vi "Frame.Export.vi"(8 "error in (no error)":errorcluster, 11 "Item Ref in":T1 format="%.0x") -> (0 "error out":errorcluster, 2 "Frame":T2 {"Signals"."Byte Order" items=["Little Endian", "Big Endian"]; "Signals"."Data Type" items=["Signed", "Unsigned", "IEEE Float"]}, 3 "Item Ref out":T1 format="%.0x")   [LabVIEW 2015, in "Diagnostics Addon System Explorer.lvlib"]
uses:
  Diagnostics Addon System Explorer.lvlib
  Types/Frame.Export.ctl
  Shared/Types/Signal.ctl
  <vilib>/NI Veristand/Custom Device API/Custom Device Item Ref.ctl
  Types/FG.Action.ctl
  Signal.FG.vi
  <vilib>/NI Veristand/Custom Device API/NI VeriStand - Get Custom Device Channel Data.vi
  <vilib>/NI Veristand/Custom Device API/NI VeriStand - Get Item Property.vi
  <vilib>/NI Veristand/Custom Device API/Get Item Property (String).vi
  <vilib>/NI Veristand/Custom Device API/Get Item Property (Double).vi
  <vilib>/NI Veristand/Custom Device API/Get Item Property (U32).vi
  <vilib>/NI Veristand/Custom Device API/NI VeriStand - Set Item Property.vi
  <vilib>/NI Veristand/Custom Device API/Set Item Property (String).vi
  <vilib>/NI Veristand/Custom Device API/Set Item Property (Double).vi
  <vilib>/NI Veristand/Custom Device API/Set Item Property (U32).vi
  Shared/SubVIs/Constants.vi
  <vilib>/NI Veristand/Custom Device API/NI VeriStand - Get Item Children.vi
  <vilib>/NI Veristand/Custom Device API/Custom Device API.lvlib
  Shared/Diagnostics Addon Shared.lvlib
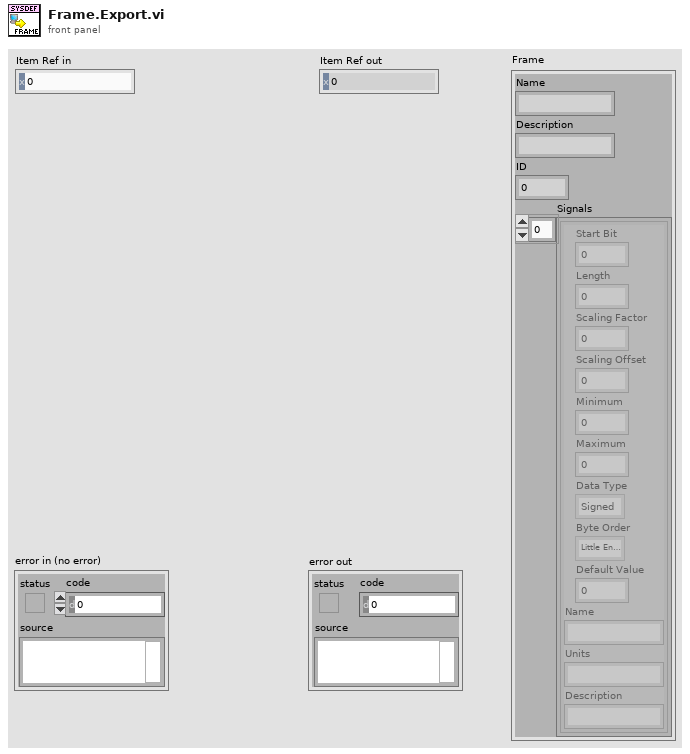
[diagram p1: front panel]
types:
  T1 = typedef "Custom Device API.lvlib/Custom Device Item Ref.ctl" = u64
  T2 = typedef "Diagnostics Addon System Explorer.lvlib/Frame.Export.ctl" = cluster{"Name":string, "Description":string, "ID":u32, "Signals":T3[]}
  T3 = typedef "Diagnostics Addon Shared.lvlib/Signal.ctl" = cluster{"Start Bit":u8, "Length":u8, "Scaling Factor":dbl, "Scaling Offset":dbl, "Minimum":dbl, "Maximum":dbl, "Data Type":u32, "Byte Order":u32, "Default Value":dbl, "Name":string, "Units":string, "Description":string}
  T4 = typedef "Diagnostics Addon System Explorer.lvlib/FG.Action.ctl" = enum16{"Get", "Set"}
  T5 = typedef "Custom Device API.lvlib/Custom Device Item Info.ctl" = cluster{"Name":string, "Is Channel":bool, "GUID":string, "Is Waveform":bool}
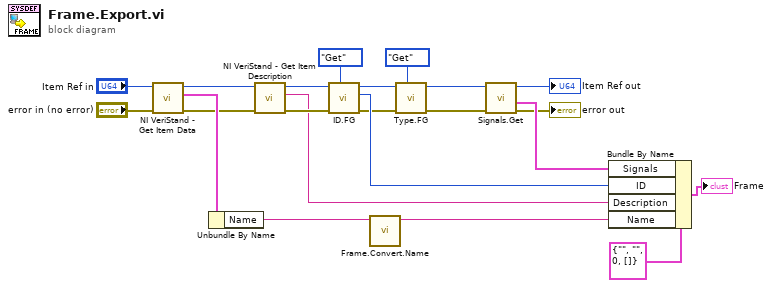
[diagram p0: block diagram]
diagram:
  n1 = call <vilib>:"NI VeriStand - Get Item Data.vi"("error in (no error)"="error in (no error)", "Item Ref in"="Item Ref in") -> ("error out"=w7:errorcluster, "Item Info"=w22:T5, "Item Ref out"=w6:T1)  [unwired: 7 out]
  n2 = Unbundle By Name(w22) -> ("Name"=w2:string)
  n3 = call <vilib>:"NI VeriStand - Get Item Description.vi"("error in (no error)"=w7, "Item Ref in"=w6) -> ("error out"=w4:errorcluster, "Description"=w3:string, "Item Ref out"=w5:T1)  [unwired: 7 out]
  n4 = call "ID.FG.vi"("Action"=FG.Action."Get", "error in (no error)"=w4, "Device Item Ref in"=w5) -> ("error out"=w10:errorcluster, "ID"=w19:u32, "Device Item Ref out"=w21:T1)  [unwired: 6 in]
  n5 = call "Frame.Convert.Name.vi"("VS Frame Name"=w2) -> ("Frame Name"=w1:string)  [unwired: 9 in, 1 out]
  n6 = call "Type.FG.vi"("Action"=FG.Action."Get", "error in (no error)"=w10, "Device Item Ref in"=w21) -> ("error out"=w9:errorcluster, "Device Item Ref out"=w11:T1)  [unwired: 6 in, 1 out]
  n7 = call "Signals.Get.vi"("error in (no error)"=w9, "Device Item Ref out"=w11) -> ("error out"=→"error out":errorcluster, "Parameters"=w18:T3[], "Item Ref out"=→"Item Ref out":T1)  [unwired: 6 in, 1 out]
  n8 = Bundle By Name(cluster=T2 {"Name"="", "Description"="", "ID"=0, "Signals"=[]} ("PID In"), "Signals"=w18, "ID"=w19, "Description"=w3, "Name"=w1) -> (→"Frame":T2)
